vi "Loop Count Global.vi"() -> ()   [LabVIEW 2012]
panel:
  out "Loop count":dbl format="%#_2f"
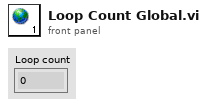
[diagram p1: front panel]
diagram:
